vi "ElevatorExecute.vi"(8 "error in (no error)":errorcluster) -> (0 "error out":errorcluster)   [LabVIEW 2023]
uses:
  <vilib>/Rock Robotics/WPI/ThirdParty/REV Robotics/REVLib/Typedef/Spark MAX Control Type.ctl
  <vilib>/Rock Robotics/WPI/ThirdParty/JAS_Junk/TrajLib/Timer_New.vi
  <vilib>/Rock Robotics/WPI/ThirdParty/REV Robotics/REVLib/SubVI/Public/SPARK Get Encoder Status Position.vi
  <vilib>/Utility/semaphor.llb/Obtain Semaphore Reference.vi
  <vilib>/Rock Robotics/WPI/ThirdParty/JAS_Junk/TrajLib/Timer_Reset.vi
  <vilib>/Rock Robotics/WPI/ThirdParty/JAS_Junk/TrajLib/Timer_Start.vi
  <vilib>/Rock Robotics/WPI/ThirdParty/JAS_Junk/TrajLib/Timer_HasPeriodPassedOnce.vi
  <vilib>/Rock Robotics/WPI/ThirdParty/JAS_Junk/TrajLib/Timer_Stop.vi
  <vilib>/Rock Robotics/WPI/ThirdParty/JAS_Junk/TrajLib/Trajectory_Library.lvlib
  <vilib>/Rock Robotics/WPI/ThirdParty/REV Robotics/REVLib/SubVI/Public/SPARK Get Limit Switch Status Forward.vi
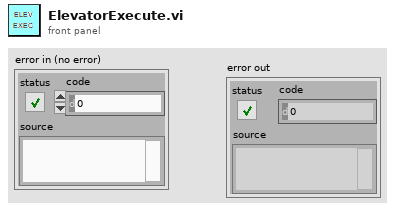
[diagram p1: front panel]
types:
  T1 = typedef "Spark MAX Control Type.ctl" = enum16{"Percent VBus", "Voltage", "Velocity", "Position", "Smart Motion", "Current", "Smart Velocity", "MAXMotion Position", "MAXMotion Velocity"}
  T2 = typedef "WPI_SwitchDevRef.ctl" = cluster{"DevStatus":errorcluster, "DIO Channel":T3, "CntIndex":T4, "Normally Closed":bool}
  T3 = typedef "FPGA_DIOChannel.ctl" = enum8{"DIO 0", "DIO 1", "DIO 2", "DIO 3", "DIO 4", "DIO 5", "DIO 6", "DIO 7", "DIO 8", "DIO 9", "DIO MXP 0", "DIO MXP 1", "DIO MXP 2", "DIO MXP 3", "DIO MXP 4", "DIO MXP 5", "DIO MXP 6", "DIO MXP 7", "DIO MXP 8", "DIO MXP 9", "DIO MXP 10", "DIO MXP 11", "DIO MXP 12", "DIO MXP 13", "DIO MXP 14", "DIO MXP 15", "SPI Port CS1", "SPI Port CS2", "SPI Port CS3", "SPI Port MISO", "SPI Port MOSI", "Invalid"}
  T4 = typedef "FPGA_CounterCtrSystemIndex.ctl" = enum8{"Ctr 0", "Ctr 1", "Ctr 2", "Ctr 3", "Ctr 4", "Ctr 5", "Ctr 6", "Ctr 7", "Invalid"}
  T5 = typedef "WPI_MotorControlDeviceRef.ctl" = cluster{"DeviceStatus":errorcluster, "Type":T6, "PWM":cluster{"PWM Channel":T7, "DeadBand":T8}, "CAN":cluster{"Device Number":u8, "SetOutput VI Ref":variant, "GetOutput VI Ref":variant, "Enable VI Ref":variant, "Disable VI Ref":variant, "Data":variant}, "Invert":bool, "DIO PWM":cluster{"PWM \"Enable\" Channel":T7, "DIOChannel":T3, "PWM Rate":dbl}}
  T6 = typedef "WPI_MotorControlType.ctl" = enum16{"PWM", "CAN", "DIO PWM"}
  T7 = typedef "FPGA_DIOPWMChannel.ctl" = enum8{"PWM 0", "PWM 1", "PWM 2", "PWM 3", "PWM 4", "PWM 5", "PWM 6", "PWM 7", "PWM 8", "PWM 9", "PWM MXP 0", "PWM MXP 1", "PWM MXP 2", "PWM MXP 3", "PWM MXP 4", "PWM MXP 5", "PWM MXP 6", "PWM MXP 7", "PWM MXP 8", "PWM MXP 9", "Invalid"}
  T8 = typedef "WPI_PWMDeadband.ctl" = cluster{"Name":string, "maxPositivePwm":i32, "minPositivePwm":i32, "centerPwm":i32, "maxNegativePwm":i32, "minNegativePwm":i32, "angularRange":u16}
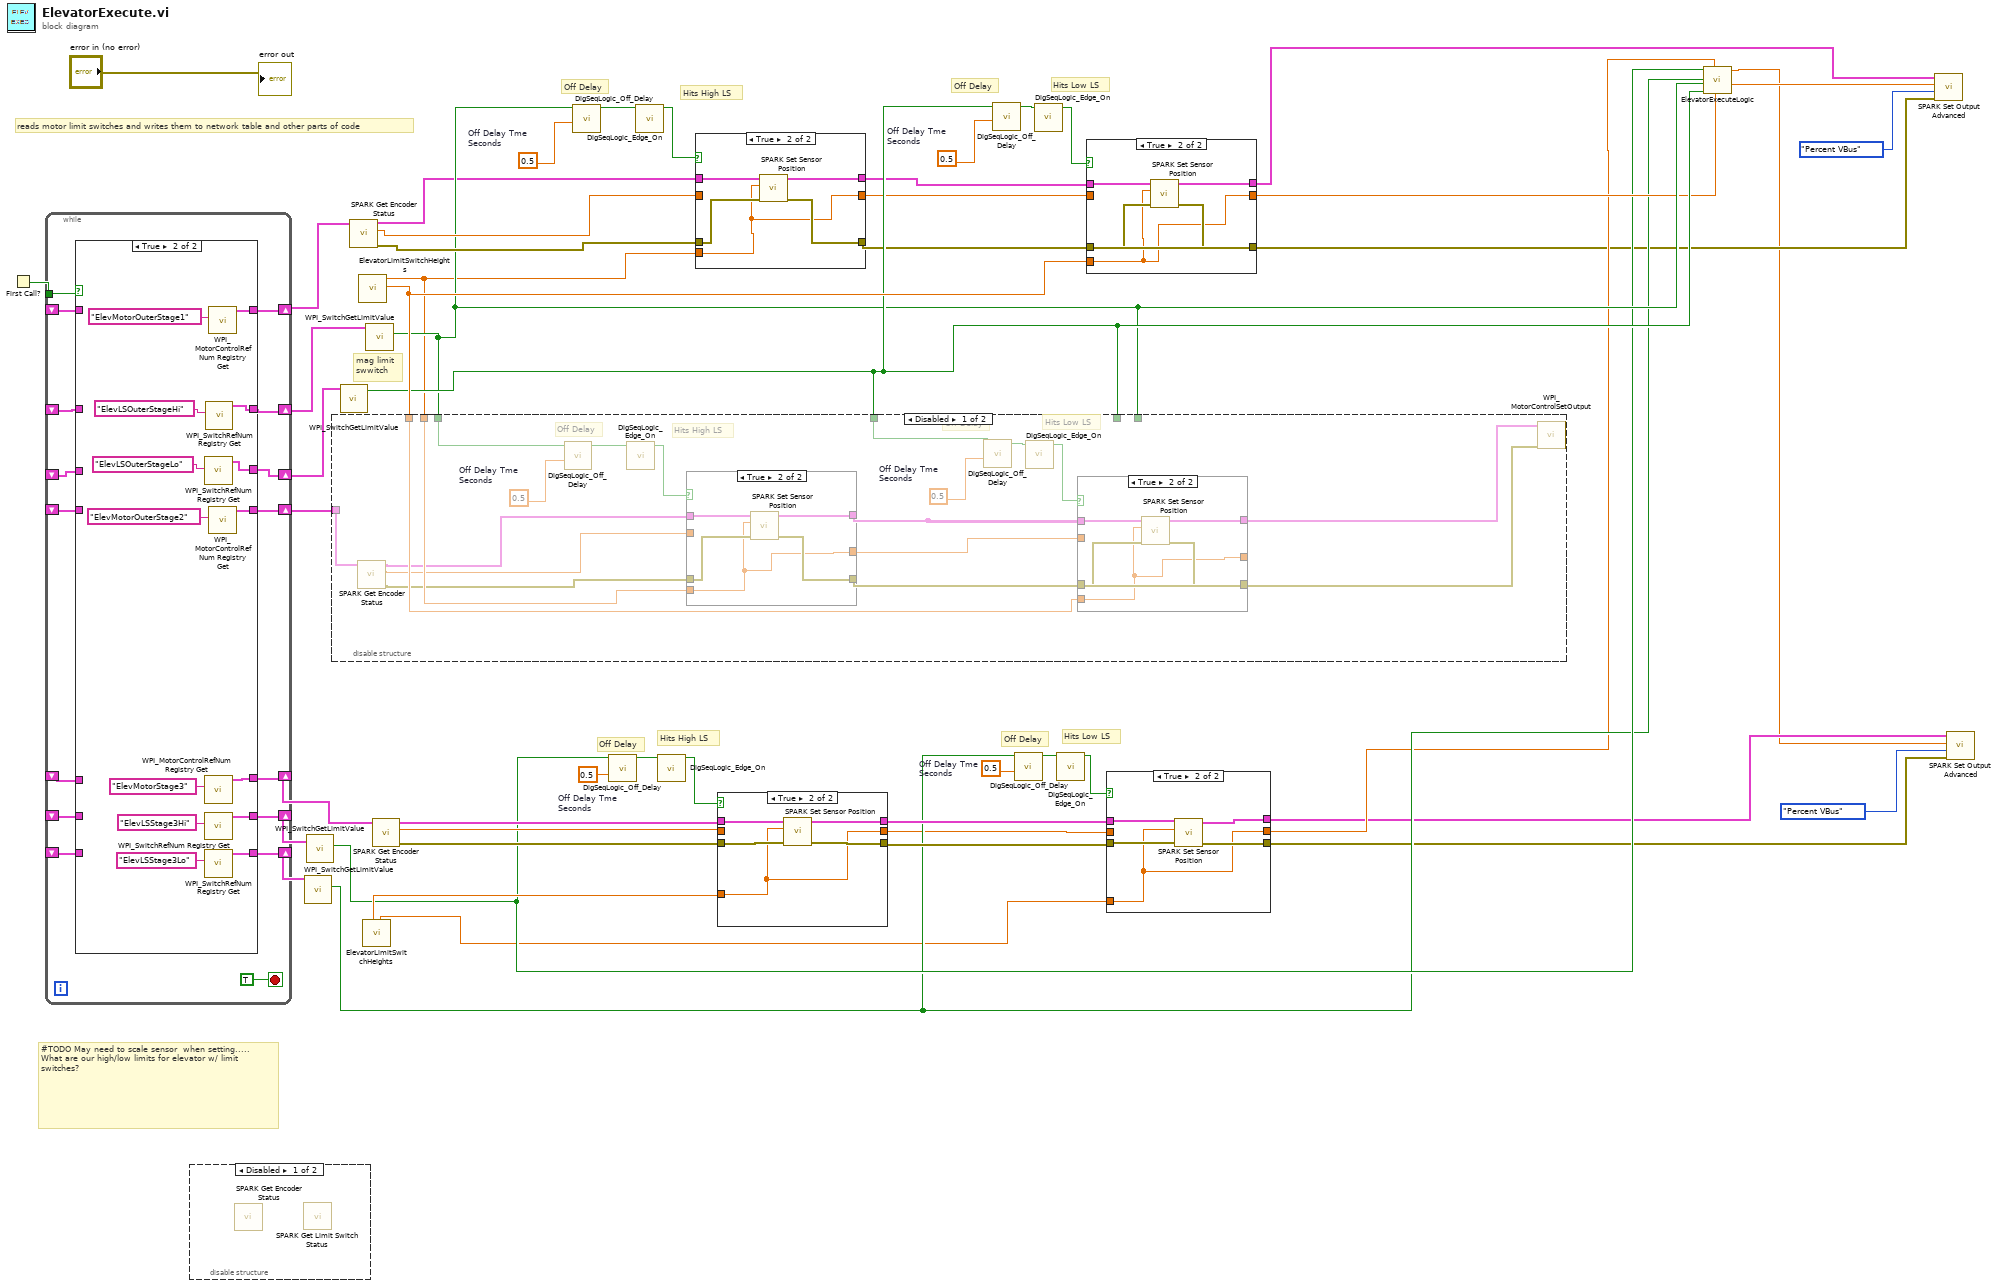
[diagram p0: block diagram]
diagram:
  w33 = 0.5  # Off Delay Tme Seconds
  w34 = 0.5  # Off Delay Tme Seconds
  w44 = 0.5  # Off Delay Tme Seconds
  w47 = 0.5  # Off Delay Tme Seconds
  # "Hits Low LS"
  # "Hits High LS"
  # "Off Delay"
  # "Off Delay"
  # "Hits Low LS"
  # "Hits High LS"
  # "Off Delay"
  # "#TODO May need to scale sensor  when setting.....\nWhat are our high/low limits for elevator w/ limit switches?"
  # "Off Delay"
  # "mag limit\nswwitch"
  # "reads motor limit switches and writes them to network table and other parts of code"
  n1 = First Call?() -> (First Call?: T/F=w48:bool)
  n2 = while {
    tunnel: w48 -> [w65]
    shift-right: [w66] -> w39
    shift-left: _ -> [w63]
    shift-right: [w62] -> w46
    shift-left: _ -> [w61]
    shift-right: [w60] -> w42
    shift-left: _ -> [w59]
    shift-right: [w58] -> w36
    shift-left: _ -> [w57]
    shift-right: [w56] -> w27
    shift-left: _ -> [w55]
    shift-right: [w54] -> w26
    shift-left: _ -> [w52]
    shift-right: [w53] -> w25
    shift-left: _ -> [w51]
    stop <- TRUE stop-if-true
    n3 = case shown="True" w65 {
      tunnel: [w73 w87] -> w66
      tunnel: w63 -> [w73 _]
      tunnel: [w72 w85] -> w62
      tunnel: w61 -> [w72 _]
      tunnel: [w71 w81] -> w60
      tunnel: w59 -> [w71 _]
      tunnel: [w70 w80] -> w58
      tunnel: w57 -> [w70 _]
      tunnel: [w69 w76] -> w56
      tunnel: w55 -> [w69 _]
      tunnel: [w68 w75] -> w54
      tunnel: [w67 w74] -> w53
      tunnel: w52 -> [w68 _]
      tunnel: w51 -> [w67 _]
      frame False {
      }
      frame True {
        n4 = call <vilib>:"WPI_SwitchRefNum Registry Get.vi"("refnum name"="ElevLSOuterStageLo") -> ("SwitchDevRef"=w81:T2)  [unwired: 9 in, 1 out]
        n5 = call <vilib>:"WPI_MotorControlRefNum Registry Get.vi"("refnum name"="ElevMotorStage3") -> ("MotorControlDevRef"=w76:T5)  [unwired: 9 in, 1 out]
        n6 = call <vilib>:"WPI_SwitchRefNum Registry Get.vi"("refnum name"="ElevLSStage3Hi") -> ("SwitchDevRef"=w75:T2)  [unwired: 9 in, 1 out]
        n7 = call <vilib>:"WPI_SwitchRefNum Registry Get.vi"("refnum name"="ElevLSStage3Lo") -> ("SwitchDevRef"=w74:T2)  [unwired: 9 in, 1 out]
        n8 = call <vilib>:"WPI_SwitchRefNum Registry Get.vi"("refnum name"="ElevLSOuterStageHi") -> ("SwitchDevRef"=w85:T2)  [unwired: 9 in, 1 out]
        n9 = call <vilib>:"WPI_MotorControlRefNum Registry Get.vi"("refnum name"="ElevMotorOuterStage1") -> ("MotorControlDevRef"=w87:T5)  [unwired: 9 in, 1 out]
        n10 = call <vilib>:"WPI_MotorControlRefNum Registry Get.vi"("refnum name"="ElevMotorOuterStage2") -> ("MotorControlDevRef"=w80:T5)  [unwired: 9 in, 1 out]
      }
    }
  }
  n11 = disable-structure shown="Disabled" {
    frame Disabled {
      n12 = call-poly <vilib>:"SPARK Get Encoder Status.vi"() -> ()  [unwired: 8 in, 4 out]
      n13 = call-poly <vilib>:"SPARK Get Limit Switch Status.vi"() -> ()  [unwired: 8 in, 4 out]
    }
    frame Enabled {
    }
  }
  n14 = call <vilib>:"WPI_SwitchGetLimitValue.vi"("SwitchDevRef"=w25) -> ("Switch Pressed"=w12:bool)  [unwired: 8 in, 2 out]
  n15 = call <vilib>:"WPI_SwitchGetLimitValue.vi"("SwitchDevRef"=w26) -> ("Switch Pressed"=w13:bool)  [unwired: 8 in, 2 out]
  n16 = call <vilib>:"WPI_SwitchGetLimitValue.vi"("SwitchDevRef"=w42) -> ("Switch Pressed"=w20:bool)  [unwired: 8 in, 2 out]
  n17 = call-poly <vilib>:"SPARK Get Encoder Status.vi"("MotorControlDevRef in"=w39) -> ("error out"=w37:errorcluster, "Sensor Position"=w38:dbl, "MotorControlDevRef out"=w17:T5)  [unwired: 7 in, 1 out]
  n18 = call "ElevatorLimitSwitchHeights.vi"() -> ("LowOuter"=w40:dbl, "HighOuter"=w18:dbl)  [unwired: 7 in, 3 out]
  n19 = call "ElevatorLimitSwitchHeights.vi"() -> ("LowStage3"=w10:dbl, "HighStage3"=w21:dbl)  [unwired: 7 in, 3 out]
  n20 = call <vilib>:"WPI_SwitchGetLimitValue.vi"("SwitchDevRef"=w46) -> ("Switch Pressed"=w19:bool)  [unwired: 8 in, 2 out]
  n21 = disable-structure shown="Disabled" {
    disable-tunnel: w19 -> [w98 _]
    disable-tunnel: w20 -> [w97 _]
    disable-tunnel: w18 -> [w96 _]
    disable-tunnel: w40 -> [w95 _]
    disable-tunnel: w36 -> [w91 _]
    disable-tunnel: w19 -> [w89 _]
    disable-tunnel: w20 -> [w88 _]
    frame Disabled {
      w103 = 0.5  # Off Delay Tme Seconds
      w106 = 0.5  # Off Delay Tme Seconds
      # "Hits Low LS"
      # "Hits High LS"
      # "Off Delay"
      # "Off Delay"
      n22 = call-poly <vilib>:"SPARK Get Encoder Status.vi"("MotorControlDevRef in"=w91) -> ("error out"=w92:errorcluster, "Sensor Position"=w93:dbl, "MotorControlDevRef out"=w94:T5)  [unwired: 7 in, 1 out]
      n23 = call <vilib>:"DigSeqLogic_Off_Delay.vi"("Delay"=w106, "Input"=w98) -> ("Output"=w105:bool)  [unwired: 8 in, 1 out]
      n24 = call <vilib>:"DigSeqLogic_Edge_On.vi"("Input"=w105) -> ("On Edge"=w107:bool)  [unwired: 10 in]
      n25 = case shown="True" w107 {
        tunnel: [w118 w123] -> w100
        tunnel: w94 -> [w118 w122]
        tunnel: [w117 w119] -> w90
        tunnel: w93 -> [w117 _]
        tunnel: w92 -> [w116 w121]
        tunnel: [w116 w120] -> w101
        tunnel: w96 -> [_ w119]
        frame False {
        }
        frame True {
          n26 = call <vilib>:"SPARK Set Sensor Position.vi"("error in"=w121, "Position"=w119, "MotorControlDeviceRef"=w122) -> ("error out"=w120:errorcluster, "MotorControlDeviceRef"=w123:T5)  [unwired: 7 in]
        }
      }
      n27 = call <vilib>:"DigSeqLogic_Off_Delay.vi"("Delay"=w103, "Input"=w97) -> ("Output"=w102:bool)  [unwired: 8 in, 1 out]
      n28 = call <vilib>:"DigSeqLogic_Edge_On.vi"("Input"=w102) -> ("On Edge"=w104:bool)  [unwired: 10 in]
      n29 = case shown="True" w104 {
        tunnel: [w110 w115] -> _
        tunnel: w100 -> [w110 w114]
        tunnel: [w109 w111] -> _
        tunnel: w90 -> [w109 _]
        tunnel: w101 -> [w108 w113]
        tunnel: [w108 w112] -> _
        tunnel: w95 -> [_ w111]
        frame False {
        }
        frame True {
          n30 = call <vilib>:"SPARK Set Sensor Position.vi"("error in"=w113, "Position"=w111, "MotorControlDeviceRef"=w114) -> ("error out"=w112:errorcluster, "MotorControlDeviceRef"=w115:T5)  [unwired: 7 in]
        }
      }
      n31 = call <vilib>:"WPI_MotorControlSetOutput.vi"("error in (no error)"=w101, "MotorControlDevRef"=w100) -> ("Output"=w99:dbl)  [unwired: 6 in, 3 out]
    }
    frame Enabled {
    }
  }
  n32 = call-poly <vilib>:"SPARK Get Encoder Status.vi"("MotorControlDevRef in"=w27) -> ("error out"=w28:errorcluster, "Sensor Position"=w29:dbl, "MotorControlDevRef out"=w30:T5)  [unwired: 7 in, 1 out]
  n33 = call <vilib>:"DigSeqLogic_Off_Delay.vi"("Delay"=w47, "Input"=w19) -> ("Output"=w41:bool)  [unwired: 8 in, 1 out]
  n34 = call <vilib>:"DigSeqLogic_Off_Delay.vi"("Delay"=w34, "Input"=w13) -> ("Output"=w31:bool)  [unwired: 8 in, 1 out]
  n35 = call <vilib>:"DigSeqLogic_Edge_On.vi"("Input"=w41) -> ("On Edge"=w49:bool)  [unwired: 10 in]
  n36 = call <vilib>:"DigSeqLogic_Edge_On.vi"("Input"=w31) -> ("On Edge"=w35:bool)  [unwired: 10 in]
  n37 = case shown="True" w49 {
    tunnel: [w124 w131] -> w16
    tunnel: w17 -> [w124 w130]
    tunnel: w38 -> [w125 _]
    tunnel: w37 -> [w126 w129]
    tunnel: [w126 w128] -> w6
    tunnel: w18 -> [_ w127]
    tunnel: [w125 w127] -> w15
    frame False {
    }
    frame True {
      n38 = call <vilib>:"SPARK Set Sensor Position.vi"("error in"=w129, "Position"=w127, "MotorControlDeviceRef"=w130) -> ("error out"=w128:errorcluster, "MotorControlDeviceRef"=w131:T5)  [unwired: 7 in]
    }
  }
  n39 = case shown="True" w35 {
    tunnel: [w134 w139] -> w24
    tunnel: w30 -> [w134 w138]
    tunnel: [w133 w135] -> w11
    tunnel: w29 -> [w133 _]
    tunnel: w28 -> [w132 w137]
    tunnel: [w132 w136] -> w23
    tunnel: w21 -> [_ w135]
    frame False {
    }
    frame True {
      n40 = call <vilib>:"SPARK Set Sensor Position.vi"("error in"=w137, "Position"=w135, "MotorControlDeviceRef"=w138) -> ("error out"=w136:errorcluster, "MotorControlDeviceRef"=w139:T5)  [unwired: 7 in]
    }
  }
  n41 = call <vilib>:"DigSeqLogic_Off_Delay.vi"("Delay"=w44, "Input"=w20) -> ("Output"=w43:bool)  [unwired: 8 in, 1 out]
  n42 = call <vilib>:"DigSeqLogic_Off_Delay.vi"("Delay"=w33, "Input"=w12) -> ("Output"=w32:bool)  [unwired: 8 in, 1 out]
  n43 = call <vilib>:"DigSeqLogic_Edge_On.vi"("Input"=w43) -> ("On Edge"=w45:bool)  [unwired: 10 in]
  n44 = call <vilib>:"DigSeqLogic_Edge_On.vi"("Input"=w32) -> ("On Edge"=w22:bool)  [unwired: 10 in]
  n45 = case shown="True" w45 {
    tunnel: [w142 w147] -> w8
    tunnel: w16 -> [w142 w146]
    tunnel: w6 -> [w141 w145]
    tunnel: [w141 w144] -> _
    tunnel: w40 -> [_ w143]
    tunnel: w15 -> [w140 _]
    tunnel: [w140 w143] -> w14
    frame False {
    }
    frame True {
      n46 = call <vilib>:"SPARK Set Sensor Position.vi"("error in"=w145, "Position"=w143, "MotorControlDeviceRef"=w146) -> ("error out"=w144:errorcluster, "MotorControlDeviceRef"=w147:T5)  [unwired: 7 in]
    }
  }
  n47 = case shown="True" w22 {
    tunnel: w24 -> [w150 w155]
    tunnel: [w150 w154] -> w3
    tunnel: w23 -> [w149 w153]
    tunnel: [w149 w152] -> w4
    tunnel: w11 -> [w148 _]
    tunnel: w10 -> [_ w151]
    tunnel: [w148 w151] -> w9
    frame False {
    }
    frame True {
      n48 = call <vilib>:"SPARK Set Sensor Position.vi"("error in"=w153, "Position"=w151, "MotorControlDeviceRef"=w155) -> ("error out"=w152:errorcluster, "MotorControlDeviceRef"=w154:T5)  [unwired: 7 in]
    }
  }
  n49 = call "ElevatorExecuteLogic.vi"("OuterPositionHeight"=w14, "InnerPositionHeight"=w9, "OuterLowLimitSwitch"=w20, "OuterHighLimitSwitch"=w19, "Stage3LowLimitSwitch"=w12, "Stage3HighLimitSwitch"=w13) -> ("OuterMotorDemand"=w7:dbl, "Stage3MotorDemand"=w2:dbl)  [unwired: 4 in]
  n50 = call <vilib>:"SPARK Set Output Advanced.vi"("error in (no error)"=w6, "Control Mode"=Spark_MAX_Control_Type."Percent VBus", "Setpoint"=w7, "MotorControlDevRef"=w8) -> ()  [unwired: 6 in, 2 out]
  n51 = call <vilib>:"SPARK Set Output Advanced.vi"("error in (no error)"=w4, "Control Mode"=Spark_MAX_Control_Type."Percent VBus", "Setpoint"=w2, "MotorControlDevRef"=w3) -> ()  [unwired: 6 in, 2 out]
  "error out" <- "error in (no error)"
